vi "Change Endianness (1D U32).vi"(11 "array in":u32[](array[numeric])) -> (3 "byte-reversed array out":u32[](array[numeric]))   [LabVIEW 2016, in "GE 5565PIORC Old.lvclass"]
uses:
  GE 5565PIORC Old.lvclass
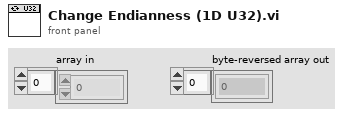
[diagram p1: front panel]
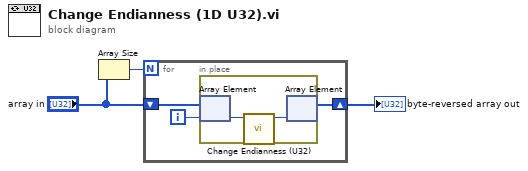
[diagram p0: block diagram]
diagram:
  n1 = Array Size(array="array in") -> (size(s)=w2:i32)
  n2 = for {
    N: w2 -> [_]
    shift-right: [w4] -> w1
    shift-left: "array in" -> [w5]
    i -> [w6]
    n3 = in-place {
      n4 = in-place-array #1(w5, w6) -> (w8:u32)
      n5 = call "Change Endianness (U32).vi"("number in"=w8) -> ("byte-reversed number out"=w7:u32)  [unwired: 10 in]
      n6 = in-place-array #1(w7) -> (w4:u32[])  [unwired: 1 out]
    }
  }
  "byte-reversed array out" <- w1
